vi "FinalProject_LastMinuteStuff.vi"() -> ()   [LabVIEW 2016]
uses:
  <vilib>/NXT/Block Support/NXT_TimerIndex.ctl
  <vilib>/NXT/Block Support/NXT_OutputPort.ctl
  <vilib>/NXT/Subs/ColorSensorColors.ctl
  <vilib>/NXT/Block Support/NXT_InputPort.ctl
  <vilib>/NXT/Dual Mode Library/Sensors/EV3_Color_Color.vi
  <vilib>/NXT/NXTIO Xnodes/NXTIONodeSubVIs/NXTMoveMotors.vi
  <vilib>/NXT/NXTIO Xnodes/NXTIONodeSubVIs/NXTStopMotors.vi
  <vilib>/NXT/NXTIO Xnodes/NXTIONodeSubVIs/NXTMotorRunDistance.vi
  <vilib>/NXT/Dual Mode Library/Sensors/EV3_Color_Reflect.vi
  <vilib>/NXT/Dual Mode Library/Waits/Wait_Num.vi
  <vilib>/NXT/Dual Mode Library/Sensors/Read_Timer.vi
  <vilib>/NXT/Dual Mode Library/Sensors/EV3_Color_RGB.vi
  <vilib>/NXT/Dual Mode Library/Sound/Tone.vi
  <vilib>/NXT/NXTIO Xnodes/AddressXNode/NXTIOAddress.xnode
  <vilib>/NXT/NXTIO Xnodes/NXTIOXNode/NXTIO.xnode
  <vilib>/NXT/Subs/LVHSConnector.ctl
  <vilib>/NXT/LegoClasses/BrickReference/BrickReference.lvclass
panel:
  out "Numeric 3":dbl
  out "Numeric 2":dbl
  out "Numeric":u32
  out "Process stopped":bool
  out "Red Large":i32
  out "Red Small":i32
  out "Blue Large":i32
  out "Blue Small":i32
  out "White Large":i32
  out "White Small":i32
  out "Steel":i32
  out "HDPE":i32
  out "Trash":i32
  out "1 Dose Small Pellets":i32
  out "1 Dose Large Pellets":i32
  out "Pellet Type":i32
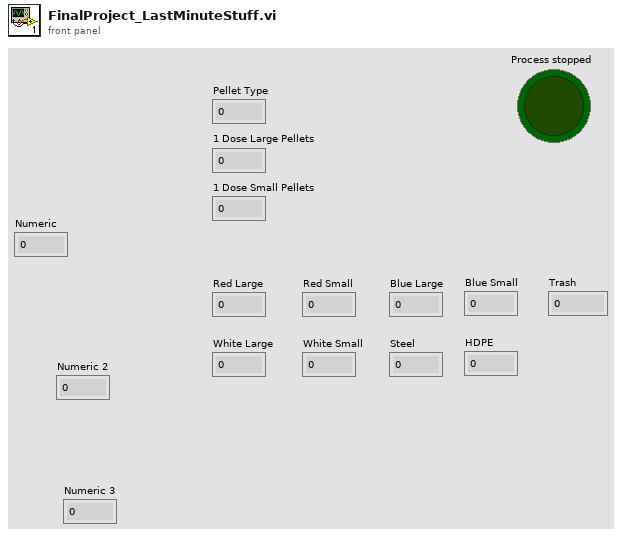
[diagram p1: front panel]
types:
  T1 = typedef "NXT_TimerIndex.ctl" = u8
  T2 = typedef "ColorSensorColors.ctl" = enum16{"No Color", "Black", "Blue", "Green", "Yellow", "Red", "White", "Brown"}
  T3 = typedef "NXT_InputPort.ctl" = u32
  T4 = typedef "NXT_OutputPort.ctl" = u8
  T5 = typedef "LVHSConnector.ctl" = refnum<class "BrickReference.lvclass">
  T6 = cluster{bool, bool, bool, bool, bool, bool, bool, bool}
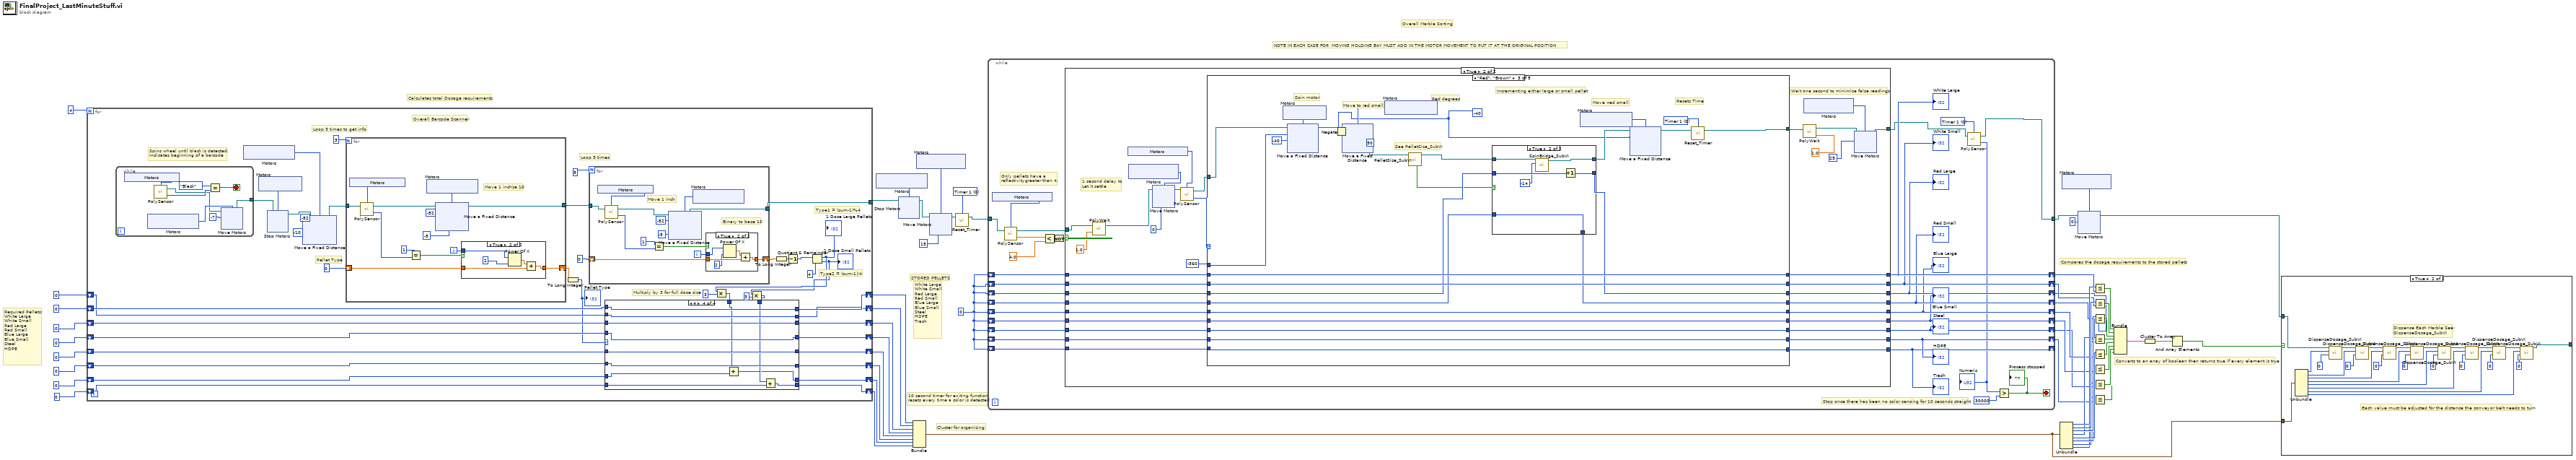
[diagram p0: block diagram]
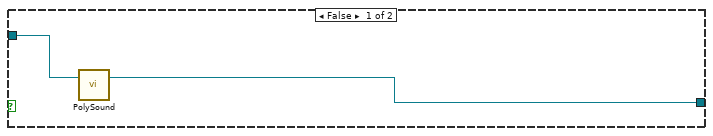
[diagram p2: hidden frame]
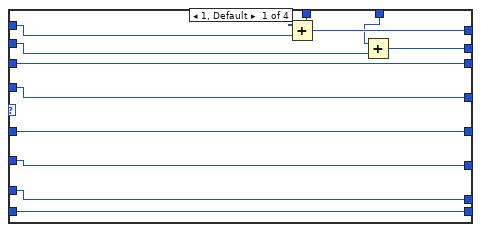
[diagram p3: hidden frame]
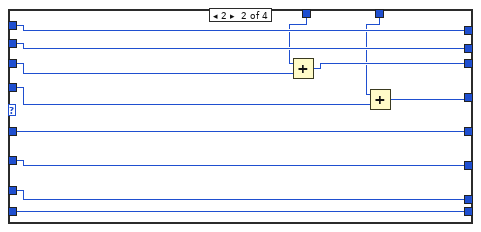
[diagram p4: hidden frame]
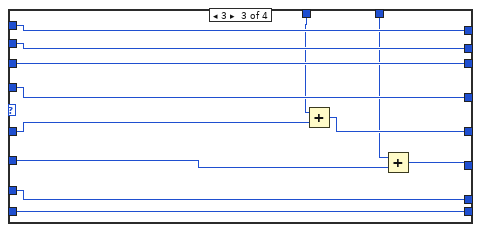
[diagram p5: hidden frame]
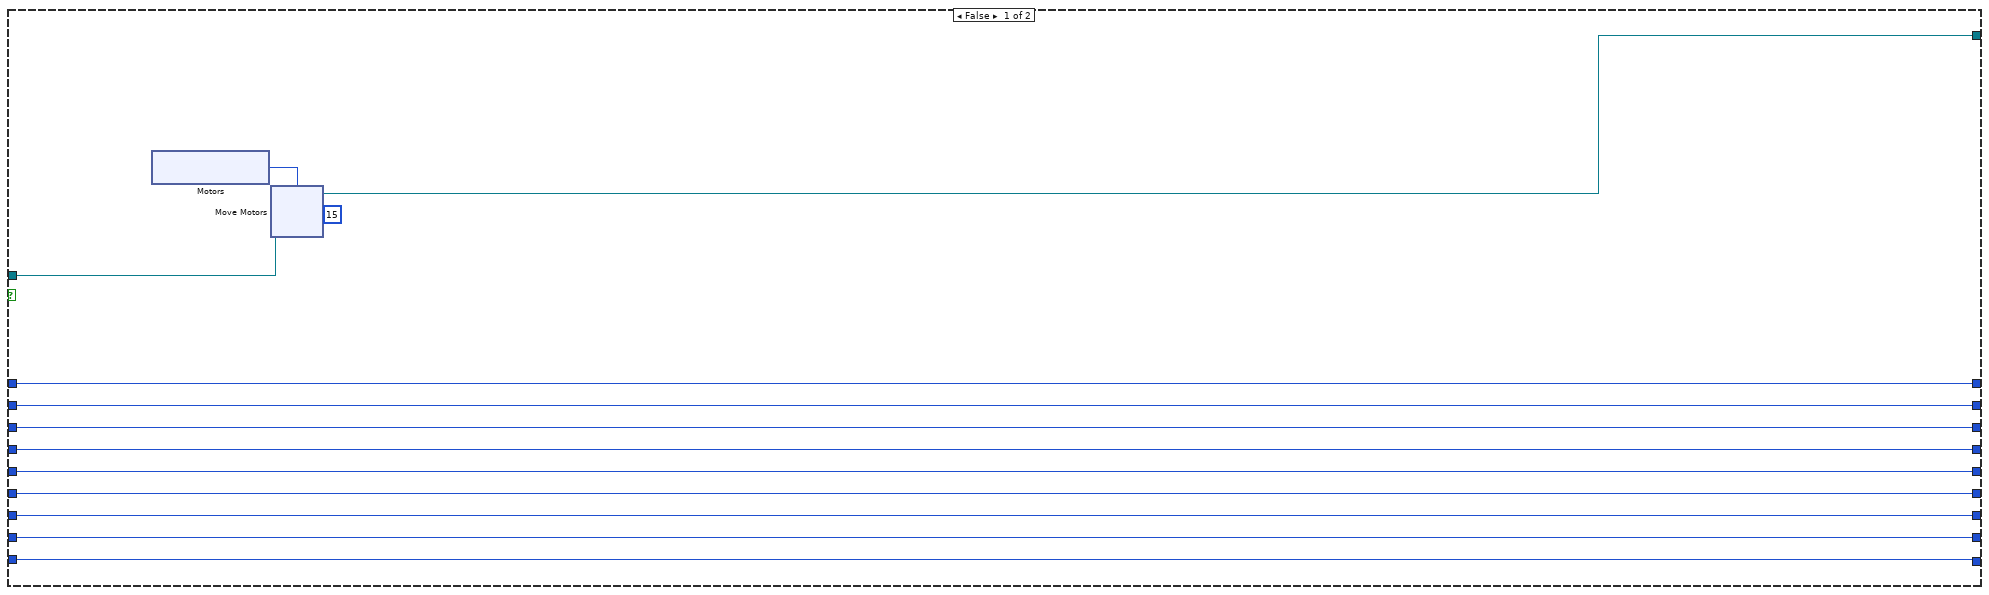
[diagram p8: hidden frame]
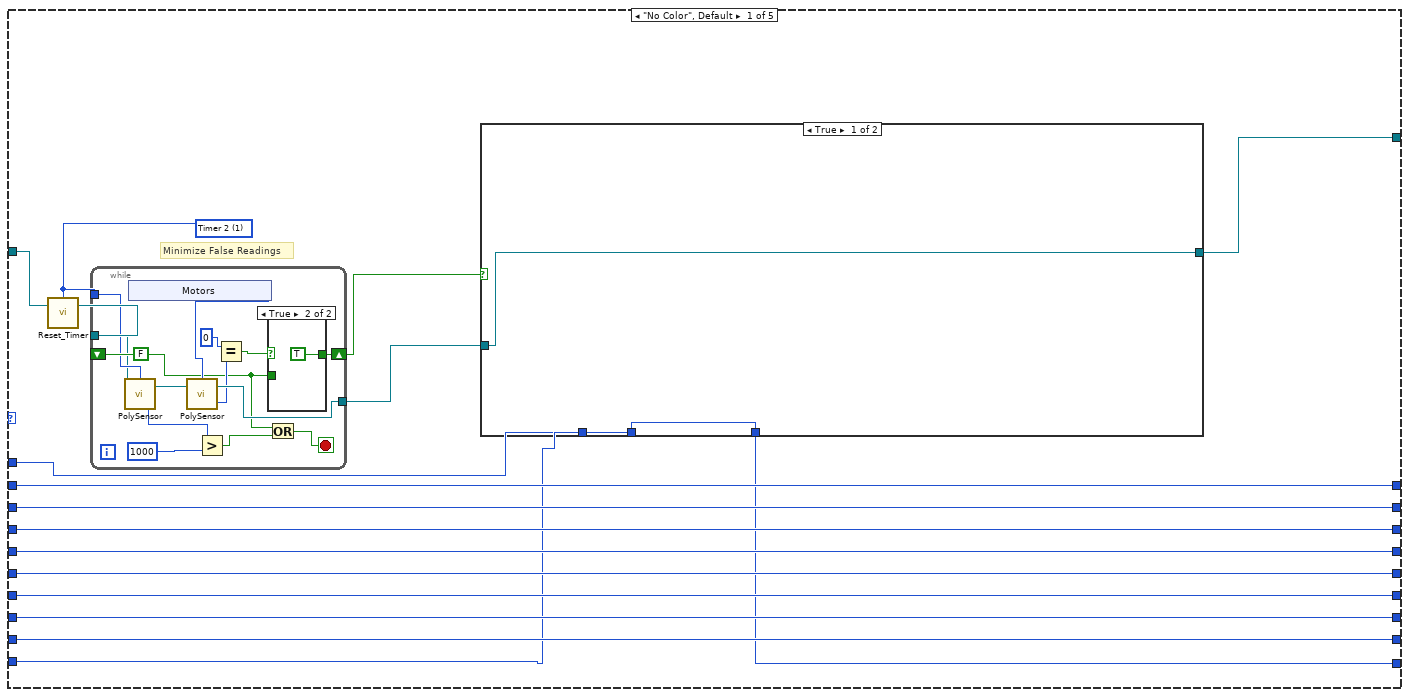
[diagram p9: hidden frame]
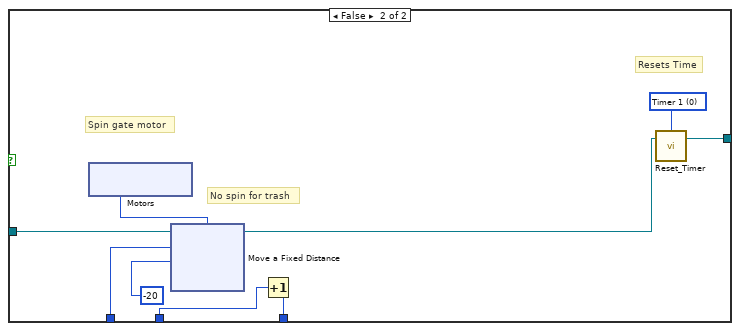
[diagram p10: hidden frame]
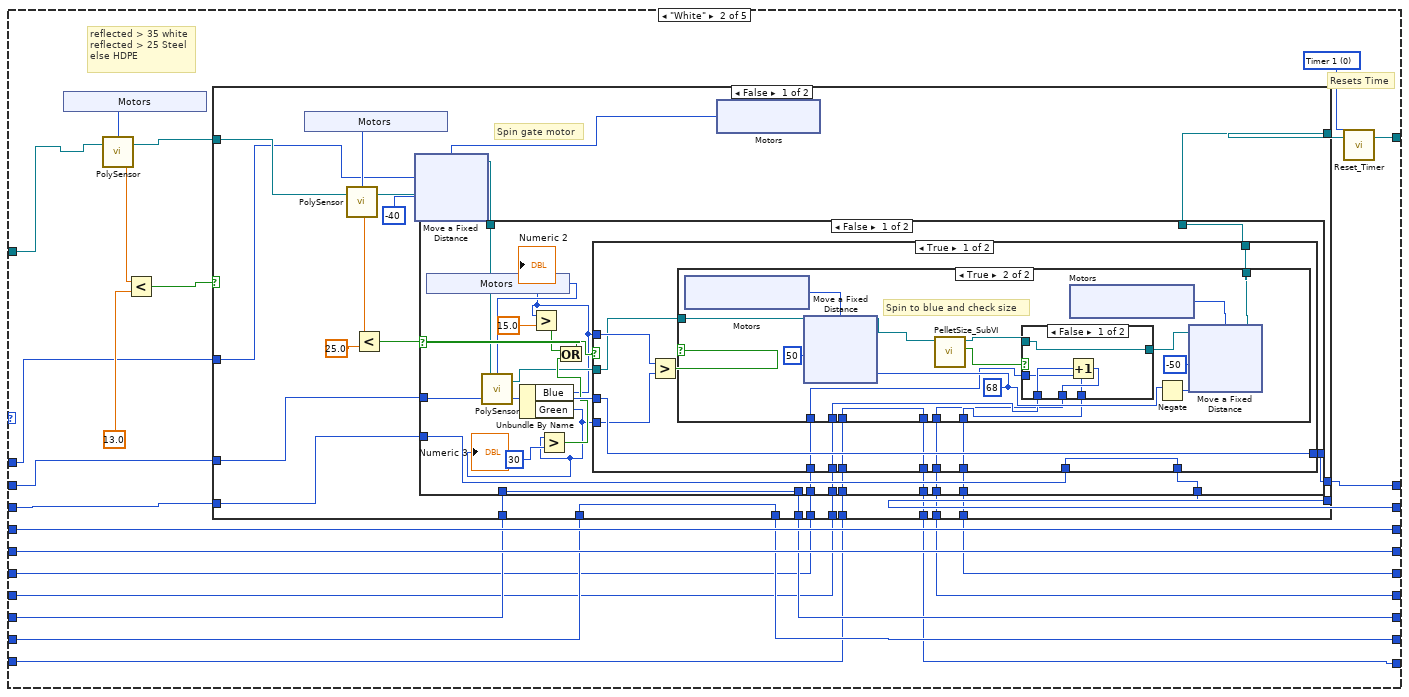
[diagram p12: hidden frame]
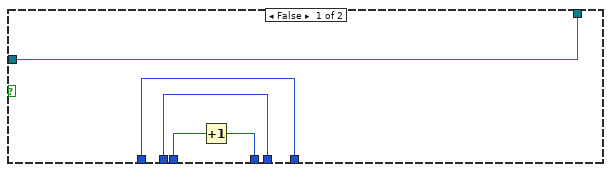
[diagram p13: hidden frame]
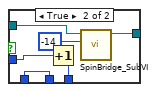
[diagram p14: hidden frame]
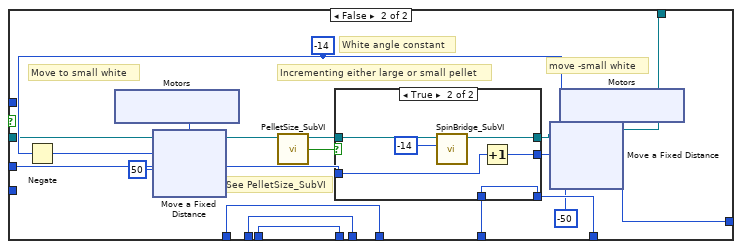
[diagram p15: hidden frame]
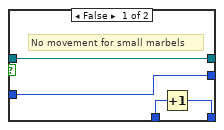
[diagram p16: hidden frame]
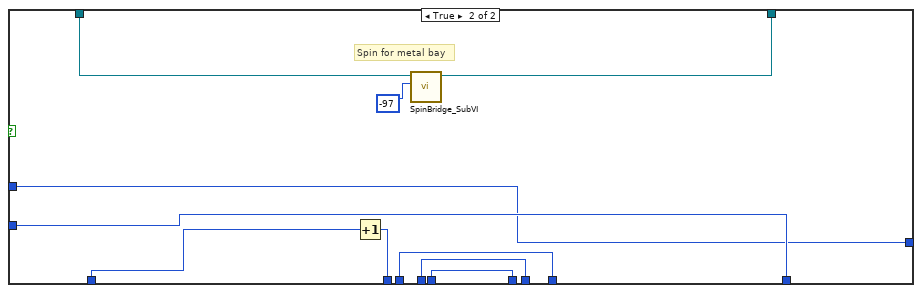
[diagram p17: hidden frame]
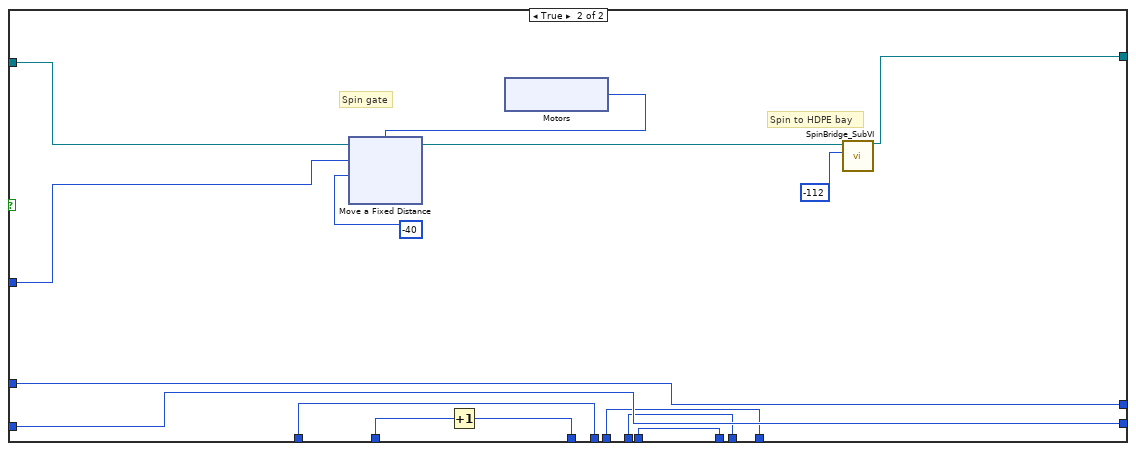
[diagram p18: hidden frame]
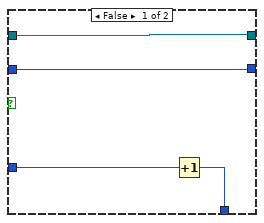
[diagram p19: hidden frame]
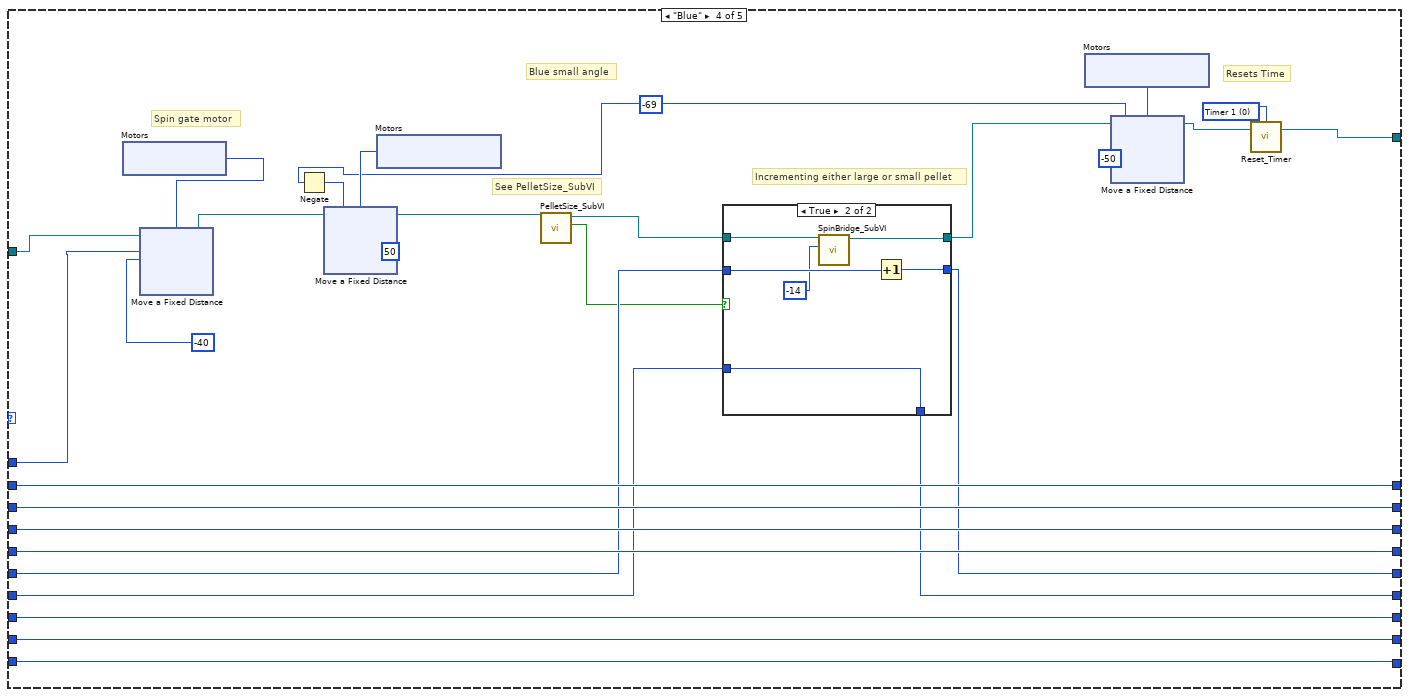
[diagram p20: hidden frame]
diagram:
  w11 = T1 0 items=["Timer 1", "Timer 2", "Timer 3"] ("Timer (Timer 1)")
  w12 = 0
  # "Cluster for organizing"
  # "Converts to an array of boolean then returns true if every element is true"
  # "Calculates total Dosage requirements"
  # "Compares the dosage requirements to the stored pellets"
  # "Required Pellets:\nWhite Large\nWhite Small\nRed Large\nRed Small\nBlue Large\nBlue Small\nSteel \nHDPE"
  # "STORED PELLETS"
  # "10 second timer for exiting function\nresets every time a color is detected"
  # "Overall Marble Sorting"
  # "NOTE IN EACH CASE FOR  MOVING HOLDING BAY MUST ADD IN THE MOTOR MOVEMENT TO PUT IT AT THE ORIGINAL POSITION"
  # "White Large\nWhite Small\nRed Large\nRed Small\nBlue Large\nBlue Small\nSteel\nHDPE\nTrash"
  n1 = for {
    N: 4 -> [_]
    tunnel: [w85] -> w14
    shift-right: [w70] -> w41
    shift-left: 0 -> [w84]
    shift-right: [w69] -> w40
    shift-left: 0 -> [w83]
    shift-right: [w76] -> w39
    shift-left: 0 -> [w82]
    shift-right: [w75] -> w38
    shift-left: 0 -> [w81]
    shift-right: [w74] -> w37
    shift-left: 0 -> [w80]
    shift-right: [w73] -> w36
    shift-left: 0 -> [w79]
    shift-right: [w72] -> w35
    shift-left: 0 -> [w78]
    shift-right: [w71] -> w17
    shift-left: 0 -> [w77]
    # "Multiply by 3 for full dose size"
    # "Overall Barcode Scanner"
    # "Spins wheel until black is detected.\nIndicates beginning of a barcode"
    # "Type2 = (sum-1)/4"
    # "Type1 = (sum-1)%4"
    # "Loop 5 times"
    # "Loop 3 times to get info"
    # "Pellet Type"
    n2 = while {
      tunnel: [w229] -> w99
      stop <- w230 stop-if-true
      n3 = xnode "Motors"() -> ("Sensor"=w227:T3)
      n4 = xnode "Motors"() -> ("Motor"=w233:T4)
      n5 = call-poly <vilib>:"PolySensor.vi"("Port (Port 1)"=w227) -> ("Detected Color"=w232:T2, "NXT/EV3"=w228:T5)  [unwired: 2 in]
      n6 = Equal?(x=ColorSensorColors."Black", y=w232) -> (x = y?=w230:bool)
      n7 = xnode "Move Motors"("Power/Speed 1"=i8 -7, "Motors"=w233, "NXT/EV3"=w228) -> ("NXT/EV3"=w229:T5)
    }
    n8 = xnode "Motors"() -> ("Motor"=w91:T4)
    n9 = xnode "Motors"() -> ("Motor"=w59:T4)
    n10 = xnode "Stop Motors"("Motors"=w59, "NXT/EV3"=w99) -> ("NXT/EV3"=w98:T5)
    n11 = xnode "Move a Fixed Distance"("Speed 1"=i8 -10, "Distance 1"=-52, "Motors"=w91, "NXT/EV3"=w98) -> ("NXT/EV3"=w96:T5)
    n12 = for {
      N: 3 -> [_]
      tunnel: w96 -> [w203]
      shift-right: [w197] -> w61
      shift-left: 0 -> [w200]
      tunnel: [w194] -> w87
      i -> [w201]
      # "Binary to base 10"
      # "Move 1 inch"
      n13 = xnode "Motors"() -> ("Sensor"=w191:T3)
      n14 = call-poly <vilib>:"PolySensor.vi"("NXT/EV3"=w203, "Port (Port 1)"=w191) -> ("Detected Color"=w202:T2, "NXT/EV3"=w199:T5)  [unwired: 1 in]
      n15 = Equal?(x=1, y=w202) -> (x = y?=w198:bool)
      n16 = xnode "Motors"() -> ("Motor"=w196:T4)
      n17 = xnode "Move a Fixed Distance"("Speed 1"=i8 -5, "Distance 1"=-52, "Motors"=w196, "NXT/EV3"=w199) -> ("NXT/EV3"=w194:T5)
      n18 = case shown="True" w198 {
        tunnel: w201 -> [_ w218]
        tunnel: w200 -> [w216 w220]
        tunnel: [w216 w219] -> w197
        frame False {
        }
        frame True {
          n19 = Power Of X(1:2, 2:w218) -> (0:w221:dbl)
          n20 = Add(x=w221, y=w220) -> (x+y=w219:dbl)
        }
      }
    }
    n21 = To Long Integer(number=w61) -> (32bit integer=w60:i32)
    "Pellet Type" <- w60
    n22 = for {
      N: 5 -> [_]
      shift-right: [w158] -> w90
      shift-left: 0 -> [w155]
      tunnel: [w157] -> w85
      tunnel: w87 -> [w156]
      i -> [w161]
      # "Binary to base 10"
      # "Move 1 inch"
      n23 = xnode "Motors"() -> ("Sensor"=w150:T3)
      n24 = call-poly <vilib>:"PolySensor.vi"("NXT/EV3"=w156, "Port (Port 1)"=w150) -> ("Detected Color"=w162:T2, "NXT/EV3"=w160:T5)  [unwired: 1 in]
      n25 = Equal?(x=1, y=w162) -> (x = y?=w159:bool)
      n26 = xnode "Motors"() -> ("Motor"=w154:T4)
      n27 = xnode "Move a Fixed Distance"("Speed 1"=i8 -5, "Distance 1"=-52, "Motors"=w154, "NXT/EV3"=w160) -> ("NXT/EV3"=w157:T5)
      n28 = case shown="True" w159 {
        tunnel: w161 -> [_ w176]
        tunnel: w155 -> [w175 w179]
        tunnel: [w175 w178] -> w158
        frame False {
        }
        frame True {
          n29 = Power Of X(1:2, 2:w176) -> (0:w180:dbl)
          n30 = Add(x=w180, y=w179) -> (x+y=w178:dbl)
        }
      }
    }
    n31 = To Long Integer(number=w90) -> (32bit integer=w89:i32)
    n32 = Decrement(x=w89) -> (x-1=w68:i32)
    n33 = Quotient & Remainder(x=w68, y=4) -> (x-y*floor(x/y)=w65:i32, floor(x/y)=w63:i32)
    "1 Dose Small Pellets" <- w63
    "1 Dose Large Pellets" <- w65
    n34 = Multiply(x=w65, y=3) -> (x*y=w64:i32)
    n35 = Multiply(x=w63, y=3) -> (x*y=w62:i32)
    n36 = case shown="4" w60 {
      tunnel: w84 -> [w105 w124 w136 w148]
      tunnel: w83 -> [w103 w123 w135 w147]
      tunnel: w82 -> [w112 w117 w134 w146]
      tunnel: w81 -> [w111 w115 w133 w145]
      tunnel: w80 -> [w110 w122 w127 w144]
      tunnel: w79 -> [w109 w121 w128 w143]
      tunnel: w78 -> [w108 w120 w126 w139]
      tunnel: w77 -> [w107 w119 w125 w138]
      tunnel: w64 -> [w106 w118 w132 w142]
      tunnel: w62 -> [w102 w114 w130 w141]
      tunnel: [w112 w116 w134 w146] -> w76
      tunnel: [w111 w113 w133 w145] -> w75
      tunnel: [w110 w122 w131 w144] -> w74
      tunnel: [w109 w121 w129 w143] -> w73
      tunnel: [w108 w120 w126 w140] -> w72
      tunnel: [w107 w119 w125 w137] -> w71
      tunnel: [w104 w124 w136 w148] -> w70
      tunnel: [w101 w123 w135 w147] -> w69
      frame 1, Default {
        n37 = Add(x=w106, y=w105) -> (x+y=w104:i32)
        n38 = Add(x=w102, y=w103) -> (x+y=w101:i32)
      }
      frame 2 {
        n39 = Add(x=w118, y=w117) -> (x+y=w116:i32)
        n40 = Add(x=w114, y=w115) -> (x+y=w113:i32)
      }
      frame 3 {
        n41 = Add(x=w132, y=w127) -> (x+y=w131:i32)
        n42 = Add(x=w130, y=w128) -> (x+y=w129:i32)
      }
      frame 4 {
        n43 = Add(x=w142, y=w139) -> (x+y=w140:i32)
        n44 = Add(x=w141, y=w138) -> (x+y=w137:i32)
      }
    }
  }
  n45 = xnode "Motors"() -> ("Motor"=w13:T4)
  n46 = xnode "Stop Motors"("Motors"=w13, "NXT/EV3"=w14) -> ("NXT/EV3"=w8:T5)
  n47 = Bundle(w41, w40, w39, w38, w37, w36, w35, w17) -> (w10:cluster{i32, i32, i32, i32, i32, i32, i32, i32})  [unwired: 1 in]
  n48 = xnode "Motors"() -> ("Motor"=w9:T4)
  n49 = xnode "Move Motors"("Power/Speed 1"=i8 15, "Motors"=w9, "NXT/EV3"=w8) -> ("NXT/EV3"=w7:T5)
  n50 = call <vilib>:"Reset_Timer.vi"("NXT/EV3"=w7, "Timer (Timer 1)"=w11) -> ("NXT/EV3"=w5:T5)  [unwired: 2 in]
  n51 = while {
    shift-right: [w260] -> w26
    shift-left: w12 -> [w269]
    shift-right: [w259] -> w25
    shift-left: w12 -> [w268]
    shift-right: [w258] -> w24
    shift-left: w12 -> [w267]
    shift-right: [w257] -> w23
    shift-left: w12 -> [w266]
    shift-right: [w254] -> w22
    shift-left: w12 -> [w265]
    shift-right: [w253] -> w21
    shift-left: w12 -> [w264]
    shift-right: [w252] -> w20
    shift-left: w12 -> [w263]
    shift-right: [w256] -> w19
    shift-left: w12 -> [w262]
    shift-right: [w255] -> _
    shift-left: w12 -> [w261]
    tunnel: w5 -> [w245]
    tunnel: [w244] -> w3
    stop <- w249 stop-if-true
    w247 = T1 0 items=["Timer 1", "Timer 2", "Timer 3"] ("Timer (Timer 1)")
    # "Stop once there has been no color sensing for 10 seconds straight"
    # "Only pellets have a\nreflectivitygreater than 4."
    n52 = xnode "Motors"() -> ("Sensor"=w251:T3)
    n53 = call-poly <vilib>:"PolySensor.vi"("NXT/EV3"=w245, "Port (Port 1)"=w251) -> ("Scaled Value"=w274:sgl, "NXT/EV3"=w270:T5)  [unwired: 1 in]
    n54 = Less?(x=w274, y=sgl 4.0) -> (x < y?=w273:bool)
    n55 = Not(x=w273) -> (.not. x?=w271:bool)
    n56 = case shown="True" w271 {
      tunnel: w270 -> [w277 w305]
      tunnel: w269 -> [w288 w329]
      tunnel: w268 -> [w287 w328]
      tunnel: w267 -> [w286 w327]
      tunnel: w266 -> [w285 w326]
      tunnel: w265 -> [w284 w325]
      tunnel: w264 -> [w283 w324]
      tunnel: w263 -> [w282 w323]
      tunnel: w262 -> [w281 w322]
      tunnel: w261 -> [w280 w321]
      tunnel: [w280 w320] -> w255
      tunnel: [w281 w318] -> w256
      tunnel: [w282 w317] -> w252
      tunnel: [w283 w316] -> w253
      tunnel: [w285 w315] -> w257
      tunnel: [w284 w314] -> w254
      tunnel: [w286 w313] -> w258
      tunnel: [w288 w312] -> w260
      tunnel: [w287 w311] -> w259
      tunnel: [w276 w300] -> w248
      frame False {
        n57 = xnode "Motors"() -> ("Motor"=w279:T4)
        n58 = xnode "Move Motors"("Power/Speed 1"=i8 15, "Motors"=w279, "NXT/EV3"=w277) -> ("NXT/EV3"=w276:T5)
      }
      frame True {
        # "Wait one second to minimize false readings"
        # "1 second delay to\nLet it settle"
        n59 = call-poly <vilib>:"PolyWait.vi"("Time (1 sec)"=sgl 1.0, "NXT/EV3"=w305) -> ("NXT/EV3"=w303:T5)  [unwired: 2 in]
        n60 = xnode "Motors"() -> ("Sensor"=w310:T3)
        n61 = xnode "Motors"() -> ("Motor"=w302:T4)
        n62 = xnode "Move Motors"("Power/Speed 1"=i8 0, "Motors"=w302, "NXT/EV3"=w303) -> ("NXT/EV3"=w307:T5)
        n63 = call-poly <vilib>:"PolySensor.vi"("NXT/EV3"=w307, "Port (Port 1)"=w310) -> ("Detected Color"=w319:T2, "NXT/EV3"=w330:T5)  [unwired: 1 in]
        n64 = case shown="\"Red\", \"Brown\"" w319 {
          tunnel: w330 -> [w352 w412 w660 w733 w794]
          tunnel: w329 -> [w359 w417 w673 w745 w803]
          tunnel: w328 -> [w358 w423 w672 w744 w802]
          tunnel: w327 -> [w360 w430 w666 w743 w801]
          tunnel: w326 -> [w362 w429 w665 w742 w800]
          tunnel: w325 -> [w361 w405 w671 w741 w799]
          tunnel: w324 -> [w363 w407 w670 w740 w798]
          tunnel: w323 -> [w364 w424 w669 w737 w797]
          tunnel: w322 -> [w365 w425 w668 w736 w806]
          tunnel: w321 -> [w350 w409 w667 w735 w807]
          tunnel: [w349 w410 w667 w735 w804] -> w320
          tunnel: [w357 w413 w649 w721 w796] -> w309
          tunnel: [w365 w422 w668 w736 w805] -> w318
          tunnel: [w364 w421 w669 w737 w797] -> w317
          tunnel: [w363 w408 w670 w738 w798] -> w316
          tunnel: [w362 w429 w663 w742 w800] -> w315
          tunnel: [w361 w406 w671 w739 w799] -> w314
          tunnel: [w360 w430 w664 w743 w801] -> w313
          tunnel: [w359 w419 w673 w745 w803] -> w312
          tunnel: [w358 w420 w672 w744 w802] -> w311
          tunnel: -360 -> [w348 w411 w646 w718 w789]
          frame "No Color", Default {
            w356 = T1 1 items=["Timer 1", "Timer 2", "Timer 3"] ("Timer (Timer 1)")
            # "Minimize False Readings"
            n65 = call <vilib>:"Reset_Timer.vi"("NXT/EV3"=w352, "Timer (Timer 1)"=w356) -> ("NXT/EV3"=w355:T5)  [unwired: 2 in]
            n66 = while {
              tunnel: w356 -> [w401]
              tunnel: w355 -> [w400]
              tunnel: [w395] -> w353
              shift-right: [w397] -> w351
              shift-left: FALSE -> [w389]
              stop <- w388 stop-if-true
              n67 = call-poly <vilib>:"PolySensor.vi"("NXT/EV3"=w400, "Timer (Timer 1)"=w401) -> ("Value (msec)"=w398:u32, "NXT/EV3"=w396:T5)  [unwired: 1 in]
              n68 = xnode "Motors"() -> ("Sensor"=w391:T3)
              n69 = call-poly <vilib>:"PolySensor.vi"("NXT/EV3"=w396, "Port (Port 1)"=w391) -> ("Detected Color"=w393:T2, "NXT/EV3"=w395:T5)  [unwired: 1 in]
              n70 = Greater?(x=w398, y=u32 1000) -> (0:w390:bool)
              n71 = Equal?(x=0, y=w393) -> (x = y?=w392:bool)
              n72 = case shown="True" w392 {
                tunnel: [w403 TRUE] -> w397
                tunnel: w389 -> [w403 _]
                frame False {
                }
                frame True {
                }
              }
              n73 = Or(x=w389, y=w390) -> (x .or. y?=w388:bool)
            }
            n74 = case shown="True" w351 {
              tunnel: [w367 w373] -> w357
              tunnel: w353 -> [w367 w371]
              tunnel: w350 -> [w366 w370]
              tunnel: [w366 w369] -> w349
              tunnel: w348 -> [_ w368]
              frame True {
              }
              frame False {
                w372 = T1 0 items=["Timer 1", "Timer 2", "Timer 3"] ("Timer (Timer 1)")
                # "Resets Time"
                # "No spin for trash"
                # "Spin gate motor"
                n75 = xnode "Motors"() -> ("Motor"=w376:T4)
                n76 = xnode "Move a Fixed Distance"("Speed 1"=i8 -20, "Distance 1"=w368, "Motors"=w376, "NXT/EV3"=w371) -> ("NXT/EV3"=w374:T5)
                n77 = Increment(x=w370) -> (x+1=w369:i32)
                n78 = call <vilib>:"Reset_Timer.vi"("NXT/EV3"=w374, "Timer (Timer 1)"=w372) -> ("NXT/EV3"=w373:T5)  [unwired: 2 in]
              }
            }
          }
          frame "White" {
            w414 = T1 0 items=["Timer 1", "Timer 2", "Timer 3"] ("Timer (Timer 1)")
            # "Resets Time"
            # "reflected > 35 white\nreflected > 25 Steel\nelse HDPE"
            n79 = xnode "Motors"() -> ("Sensor"=w416:T3)
            n80 = call-poly <vilib>:"PolySensor.vi"("NXT/EV3"=w412, "Port (Port 1)"=w416) -> ("Scaled Value"=w428:sgl, "NXT/EV3"=w418:T5)  [unwired: 1 in]
            n81 = Less?(x=w428, y=sgl 13.0) -> (x < y?=w426:bool)
            n82 = case shown="False" w426 {
              tunnel: w425 -> [w455 w634]
              tunnel: w424 -> [w453 w632]
              tunnel: w423 -> [w449 w631]
              tunnel: w417 -> [w445 w630]
              tunnel: [w455 w633] -> w422
              tunnel: [w448 w632] -> w421
              tunnel: [w447 w631] -> w420
              tunnel: [w446 w630] -> w419
              tunnel: w418 -> [w454 w627]
              tunnel: [w444 w625] -> w415
              tunnel: w411 -> [w438 w623]
              tunnel: [w437 w622] -> w410
              tunnel: w409 -> [w436 w622]
              tunnel: [w435 w621] -> w408
              tunnel: w407 -> [w434 w621]
              tunnel: [w433 w620] -> w406
              tunnel: w405 -> [w432 w620]
              frame False {
                # "Spin gate motor"
                n83 = xnode "Motors"() -> ("Sensor"=w443:T3)
                n84 = call-poly <vilib>:"PolySensor.vi"("NXT/EV3"=w454, "Port (Port 1)"=w443) -> ("Scaled Value"=w452:sgl, "NXT/EV3"=w440:T5)  [unwired: 1 in]
                n85 = Less?(x=w452, y=sgl 25.0) -> (x < y?=w450:bool)
                n86 = xnode "Motors"() -> ("Motor"=w442:T4)
                n87 = xnode "Move a Fixed Distance"("Speed 1"=i8 -40, "Distance 1"=w438, "Motors"=w442, "NXT/EV3"=w440) -> ("NXT/EV3"=w439:T5)
                n88 = case shown="False" w450 {
                  tunnel: w453 -> [w490 w616]
                  tunnel: w449 -> [w489 w618]
                  tunnel: w445 -> [w487 w617]
                  tunnel: [w490 w619] -> w448
                  tunnel: [w488 w618] -> w447
                  tunnel: [w486 w617] -> w446
                  tunnel: [w485 w614] -> w444
                  tunnel: w439 -> [w484 w615]
                  tunnel: [w480 w612] -> w437
                  tunnel: w436 -> [w479 w612]
                  tunnel: [w473 w611] -> w435
                  tunnel: w434 -> [w472 w611]
                  tunnel: [w471 w610] -> w433
                  tunnel: w432 -> [w470 w610]
                  frame False {
                    n89 = xnode "Motors"() -> ("Sensor"=w483:T3)
                    n90 = call-poly <vilib>:"PolySensor.vi"("NXT/EV3"=w484, "Port (Port 1)"=w483) -> ("RGB Color"=w482:cluster{"Red":u8, "Green":u8, "Blue":u8}, "NXT/EV3"=w474:T5)  [unwired: 1 in]
                    n91 = Unbundle By Name(w482) -> ("Blue"=w468:u8, "Green"=w469:u8)
                    "Numeric 2" <- w468
                    "Numeric 3" <- w469
                    n92 = Greater?(x=w468, y=15.0) -> (0:w477:bool)
                    n93 = Greater?(x=w469, y=30) -> (0:w476:bool)
                    n94 = Or(x=w477, y=w476) -> (x .or. y?=w475:bool)
                    n95 = case shown="True" w475 {
                      tunnel: w489 -> [w502 w576]
                      tunnel: [w502 w575] -> w488
                      tunnel: w487 -> [w503 w574]
                      tunnel: [w503 w573] -> w486
                      tunnel: [w492 w568] -> w485
                      tunnel: [w500 w561] -> w480
                      tunnel: w479 -> [w501 w561]
                      tunnel: w474 -> [w491 w560]
                      tunnel: [w499 w559] -> w473
                      tunnel: w472 -> [w498 w559]
                      tunnel: w469 -> [w497 _]
                      tunnel: w468 -> [w496 _]
                      tunnel: [w494 w558] -> w471
                      tunnel: w470 -> [w493 w558]
                      frame True {
                        n96 = Greater?(x=w496, y=w497) -> (0:w495:bool)
                        n97 = case shown="True" w495 {
                          tunnel: w501 -> [w508 w525]
                          tunnel: [w507 w525] -> w500
                          tunnel: [w506 w511] -> w499
                          tunnel: w498 -> [w506 w514]
                          tunnel: [w505 w512] -> w494
                          tunnel: w493 -> [w505 w513]
                          tunnel: [w504 w520] -> w492
                          tunnel: w491 -> [w504 w523]
                          frame False {
                            n98 = Increment(x=w508) -> (x+1=w507:i32)
                          }
                          frame True {
                            w519 = 68
                            # "Spin to blue and check size"
                            n99 = xnode "Motors"() -> ("Motor"=w522:T4)
                            n100 = xnode "Move a Fixed Distance"("Speed 1"=i8 50, "Distance 1"=w519, "Motors"=w522, "NXT/EV3"=w523) -> ("NXT/EV3"=w516:T5)
                            n101 = call "PelletSize_SubVI.vi"("BrickReference in"=w516) -> ("Boolean"=w524:bool, "BrickReference out"=w510:T5)  [unwired: 9 in]
                            n102 = case shown="False" w524 {
                              tunnel: w514 -> [w541 w545]
                              tunnel: w513 -> [w539 w547]
                              tunnel: [w539 w546] -> w512
                              tunnel: [w540 w545] -> w511
                              tunnel: w510 -> [w538 w543]
                              tunnel: [w538 w542] -> w509
                              frame False {
                                n103 = Increment(x=w541) -> (x+1=w540:i32)
                              }
                              frame True {
                                n104 = Increment(x=w547) -> (x+1=w546:i32)
                                n105 = call "SpinBridge_SubVI.vi"("Motor Spin in"=-14, "BrickReference in"=w543) -> ("BrickReference out"=w542:T5)  [unwired: 9 in]
                              }
                            }
                            n106 = xnode "Motors"() -> ("Motor"=w521:T4)
                            n107 = Negate(x=w519) -> (-x=w518:i32)
                            n108 = xnode "Move a Fixed Distance"("Speed 1"=i8 -50, "Distance 1"=w518, "Motors"=w521, "NXT/EV3"=w509) -> ("NXT/EV3"=w520:T5)
                          }
                        }
                      }
                      frame False {
                        w563 = -14
                        # "White angle constant"
                        # "move -small white"
                        # "Move to small white"
                        # "See PelletSize_SubVI"
                        # "Incrementing either large or small pellet"
                        n109 = Negate(x=w563) -> (-x=w567:i32)
                        n110 = xnode "Motors"() -> ("Motor"=w565:T4)
                        n111 = xnode "Move a Fixed Distance"("Speed 1"=i8 50, "Distance 1"=w567, "Motors"=w565, "NXT/EV3"=w560) -> ("NXT/EV3"=w570:T5)
                        n112 = call "PelletSize_SubVI.vi"("BrickReference in"=w570) -> ("Boolean"=w572:bool, "BrickReference out"=w571:T5)  [unwired: 9 in]
                        n113 = case shown="True" w572 {
                          tunnel: w576 -> [w602 w608]
                          tunnel: [w601 w608] -> w575
                          tunnel: w574 -> [w600 w607]
                          tunnel: [w600 w606] -> w573
                          tunnel: w571 -> [w599 w605]
                          tunnel: [w599 w604] -> w569
                          frame False {
                            # "No movement for small marbels"
                            n114 = Increment(x=w602) -> (x+1=w601:i32)
                          }
                          frame True {
                            n115 = call "SpinBridge_SubVI.vi"("Motor Spin in"=-14, "BrickReference in"=w605) -> ("BrickReference out"=w604:T5)  [unwired: 9 in]
                            n116 = Increment(x=w607) -> (x+1=w606:i32)
                          }
                        }
                        n117 = xnode "Motors"() -> ("Motor"=w564:T4)
                        n118 = xnode "Move a Fixed Distance"("Speed 1"=i8 -50, "Distance 1"=w563, "Motors"=w564, "NXT/EV3"=w569) -> ("NXT/EV3"=w568:T5)
                      }
                    }
                  }
                  frame True {
                    # "Spin for metal bay"
                    n119 = Increment(x=w616) -> (x+1=w619:i32)
                    n120 = call "SpinBridge_SubVI.vi"("Motor Spin in"=-97, "BrickReference in"=w615) -> ("BrickReference out"=w614:T5)  [unwired: 9 in]
                  }
                }
              }
              frame True {
                # "Spin to HDPE bay"
                # "Spin gate"
                n121 = Increment(x=w634) -> (x+1=w633:i32)
                n122 = xnode "Motors"() -> ("Motor"=w629:T4)
                n123 = xnode "Move a Fixed Distance"("Speed 1"=i8 -40, "Distance 1"=w623, "Motors"=w629, "NXT/EV3"=w627) -> ("NXT/EV3"=w626:T5)
                n124 = call "SpinBridge_SubVI.vi"("Motor Spin in"=-112, "BrickReference in"=w626) -> ("BrickReference out"=w625:T5)  [unwired: 9 in]
              }
            }
            n125 = call <vilib>:"Reset_Timer.vi"("NXT/EV3"=w415, "Timer (Timer 1)"=w414) -> ("NXT/EV3"=w413:T5)  [unwired: 2 in]
          }
          frame "Red", "Brown" {
            w648 = T1 0 items=["Timer 1", "Timer 2", "Timer 3"] ("Timer (Timer 1)")
            w647 = -40
            # "Resets Time"
            # "Red degrees"
            # "Move -red small"
            # "Move to red small"
            # "See PelletSize_SubVI"
            # "Incrementing either large or small pellet"
            # "Spin motor"
            n126 = xnode "Motors"() -> ("Motor"=w662:T4)
            n127 = xnode "Move a Fixed Distance"("Speed 1"=i8 -40, "Distance 1"=w646, "Motors"=w662, "NXT/EV3"=w660) -> ("NXT/EV3"=w656:T5)
            n128 = Negate(x=w647) -> (-x=w654:i32)
            n129 = xnode "Motors"() -> ("Motor"=w652:T4)
            n130 = xnode "Move a Fixed Distance"("Speed 1"=i8 50, "Distance 1"=w654, "Motors"=w652, "NXT/EV3"=w656) -> ("NXT/EV3"=w657:T5)
            n131 = call "PelletSize_SubVI.vi"("BrickReference in"=w657) -> ("Boolean"=w658:bool, "BrickReference out"=w659:T5)  [unwired: 9 in]
            n132 = case shown="True" w658 {
              tunnel: w666 -> [w710 w716]
              tunnel: w665 -> [w709 w714]
              tunnel: [w710 w715] -> w664
              tunnel: [w708 w714] -> w663
              tunnel: w659 -> [w707 w713]
              tunnel: [w707 w712] -> w655
              frame False {
                n133 = Increment(x=w709) -> (x+1=w708:i32)
              }
              frame True {
                n134 = call "SpinBridge_SubVI.vi"("Motor Spin in"=-14, "BrickReference in"=w713) -> ("BrickReference out"=w712:T5)  [unwired: 9 in]
                n135 = Increment(x=w716) -> (x+1=w715:i32)
              }
            }
            n136 = xnode "Motors"() -> ("Motor"=w651:T4)
            n137 = xnode "Move a Fixed Distance"("Speed 1"=w647, "Distance 1"=w647, "Motors"=w651, "NXT/EV3"=w655) -> ("NXT/EV3"=w650:T5)
            n138 = call <vilib>:"Reset_Timer.vi"("NXT/EV3"=w650, "Timer (Timer 1)"=w648) -> ("NXT/EV3"=w649:T5)  [unwired: 2 in]
          }
          frame "Blue" {
            w720 = T1 0 items=["Timer 1", "Timer 2", "Timer 3"] ("Timer (Timer 1)")
            w719 = -69
            # "Resets Time"
            # "Blue small angle"
            # "See PelletSize_SubVI"
            # "Incrementing either large or small pellet"
            # "Spin gate motor"
            n139 = xnode "Motors"() -> ("Motor"=w730:T4)
            n140 = xnode "Move a Fixed Distance"("Speed 1"=i8 -40, "Distance 1"=w718, "Motors"=w730, "NXT/EV3"=w733) -> ("NXT/EV3"=w729:T5)
            n141 = Negate(x=w719) -> (-x=w726:i32)
            n142 = xnode "Motors"() -> ("Motor"=w724:T4)
            n143 = xnode "Move a Fixed Distance"("Speed 1"=i8 50, "Distance 1"=w726, "Motors"=w724, "NXT/EV3"=w729) -> ("NXT/EV3"=w728:T5)
            n144 = call "PelletSize_SubVI.vi"("BrickReference in"=w728) -> ("Boolean"=w732:bool, "BrickReference out"=w731:T5)  [unwired: 9 in]
            n145 = case shown="True" w732 {
              tunnel: w741 -> [w782 w788]
              tunnel: w740 -> [w781 w786]
              tunnel: [w782 w787] -> w739
              tunnel: [w780 w786] -> w738
              tunnel: w731 -> [w779 w785]
              tunnel: [w779 w784] -> w727
              frame False {
                n146 = Increment(x=w781) -> (x+1=w780:i32)
              }
              frame True {
                n147 = call "SpinBridge_SubVI.vi"("Motor Spin in"=-14, "BrickReference in"=w785) -> ("BrickReference out"=w784:T5)  [unwired: 9 in]
                n148 = Increment(x=w788) -> (x+1=w787:i32)
              }
            }
            n149 = xnode "Motors"() -> ("Motor"=w723:T4)
            n150 = xnode "Move a Fixed Distance"("Speed 1"=-50, "Distance 1"=w719, "Motors"=w723, "NXT/EV3"=w727) -> ("NXT/EV3"=w722:T5)
            n151 = call <vilib>:"Reset_Timer.vi"("NXT/EV3"=w722, "Timer (Timer 1)"=w720) -> ("NXT/EV3"=w721:T5)  [unwired: 2 in]
          }
          frame "Black" {
            w795 = T1 1 items=["Timer 1", "Timer 2", "Timer 3"] ("Timer (Timer 1)")
            # "Minimize False Readings"
            n152 = call <vilib>:"Reset_Timer.vi"("NXT/EV3"=w794, "Timer (Timer 1)"=w795) -> ("NXT/EV3"=w793:T5)  [unwired: 2 in]
            n153 = while {
              tunnel: w795 -> [w821]
              tunnel: w793 -> [w820]
              tunnel: [w815] -> w792
              shift-right: [w817] -> w790
              shift-left: FALSE -> [w809]
              stop <- w808 stop-if-true
              n154 = call-poly <vilib>:"PolySensor.vi"("NXT/EV3"=w820, "Timer (Timer 1)"=w821) -> ("Value (msec)"=w818:u32, "NXT/EV3"=w816:T5)  [unwired: 1 in]
              n155 = xnode "Motors"() -> ("Sensor"=w811:T3)
              n156 = call-poly <vilib>:"PolySensor.vi"("NXT/EV3"=w816, "Port (Port 1)"=w811) -> ("Detected Color"=w813:T2, "NXT/EV3"=w815:T5)  [unwired: 1 in]
              n157 = Greater?(x=w818, y=u32 1000) -> (0:w810:bool)
              n158 = Equal?(x=0, y=w813) -> (x = y?=w812:bool)
              n159 = case shown="True" w812 {
                tunnel: [w823 TRUE] -> w817
                tunnel: w809 -> [w823 _]
                frame False {
                }
                frame True {
                }
              }
              n160 = Or(x=w809, y=w810) -> (x .or. y?=w808:bool)
            }
            n161 = case shown="False" w790 {
              tunnel: w807 -> [w838 w866]
              tunnel: w806 -> [w837 w865]
              tunnel: [w836 w865] -> w805
              tunnel: [w835 w866] -> w804
              tunnel: w792 -> [w834 w864]
              tunnel: [w827 w864] -> w796
              tunnel: w789 -> [w825 _]
              frame False {
                w826 = T1 0 items=["Timer 1", "Timer 2", "Timer 3"] ("Timer (Timer 1)")
                # "Resets Time"
                # "Determine if a trash or opaque pellet"
                # "Spin gate"
                # "if reflect > 15 HDPE\nelse trash"
                n162 = xnode "Motors"() -> ("Sensor"=w833:T3)
                n163 = call-poly <vilib>:"PolySensor.vi"("NXT/EV3"=w834, "Port (Port 1)"=w833) -> ("Scaled Value"=w840:sgl, "NXT/EV3"=w830:T5)  [unwired: 1 in]
                n164 = Greater?(x=w840, y=14.0) -> (0:w839:bool)
                n165 = xnode "Motors"() -> ("Motor"=w832:T4)
                n166 = xnode "Move a Fixed Distance"("Speed 1"=i8 -40, "Distance 1"=w825, "Motors"=w832, "NXT/EV3"=w830) -> ("NXT/EV3"=w829:T5)
                n167 = case shown="False" w839 {
                  tunnel: w838 -> [w857 w861]
                  tunnel: w837 -> [w855 w863]
                  tunnel: [w855 w862] -> w836
                  tunnel: [w856 w861] -> w835
                  tunnel: w829 -> [w854 w860]
                  tunnel: [w854 w859] -> w828
                  frame False {
                    # "No movement for trash"
                    n168 = Increment(x=w857) -> (x+1=w856:i32)
                  }
                  frame True {
                    # "Spin to opaque bay and then return"
                    n169 = Increment(x=w863) -> (x+1=w862:i32)
                    n170 = call "SpinBridge_SubVI.vi"("Motor Spin in"=-114, "BrickReference in"=w860) -> ("BrickReference out"=w859:T5)  [unwired: 9 in]
                  }
                }
                n171 = call <vilib>:"Reset_Timer.vi"("NXT/EV3"=w828, "Timer (Timer 1)"=w826) -> ("NXT/EV3"=w827:T5)  [unwired: 2 in]
              }
              frame True {
              }
            }
          }
        }
        n172 = call-poly <vilib>:"PolyWait.vi"("Time (1 sec)"=sgl 1.0, "NXT/EV3"=w309) -> ("NXT/EV3"=w298:T5)  [unwired: 2 in]
        n173 = xnode "Motors"() -> ("Motor"=w299:T4)
        n174 = xnode "Move Motors"("Power/Speed 1"=25, "Motors"=w299, "NXT/EV3"=w298) -> ("NXT/EV3"=w300:T5)
      }
    }
    "Red Large" <- w258
    "Red Small" <- w257
    "Blue Large" <- w254
    "Blue Small" <- w253
    "White Large" <- w260
    "White Small" <- w259
    "Steel" <- w252
    "HDPE" <- w256
    "Trash" <- w255
    n175 = call-poly <vilib>:"PolySensor.vi"("NXT/EV3"=w248, "Timer (Timer 1)"=w247) -> ("Value (msec)"=w246:u32, "NXT/EV3"=w244:T5)  [unwired: 1 in]
    "Numeric" <- w246
    n176 = Greater?(x=w246, y=u32 30000) -> (0:w249:bool)
    "Process stopped" <- w249
  }
  n177 = Unbundle(w10) -> (w34:i32, w33:i32, w32:i32, w31:i32, w30:i32, w29:i32, w28:i32, w27:i32)
  n178 = xnode "Motors"() -> ("Motor"=w4:T4)
  n179 = xnode "Move Motors"("Power/Speed 1"=i8 0, "Motors"=w4, "NXT/EV3"=w3) -> ("NXT/EV3"=w2:T5)
  n180 = Less Or Equal?(x=w34, y=w26) -> (x <= y?=w58:bool)
  n181 = Less Or Equal?(x=w33, y=w25) -> (x <= y?=w57:bool)
  n182 = Less Or Equal?(x=w32, y=w24) -> (x <= y?=w56:bool)
  n183 = Less Or Equal?(x=w31, y=w23) -> (x <= y?=w55:bool)
  n184 = Less Or Equal?(x=w30, y=w22) -> (x <= y?=w54:bool)
  n185 = Less Or Equal?(x=w29, y=w21) -> (x <= y?=w53:bool)
  n186 = Less Or Equal?(x=w28, y=w20) -> (x <= y?=w52:bool)
  n187 = Less Or Equal?(x=w27, y=w19) -> (x <= y?=w51:bool)
  n188 = Bundle(w58, w57, w56, w55, w54, w53, w52, w51) -> (w50:T6)  [unwired: 1 in]
  n189 = Cluster To Array(cluster=w50) -> (array=w49:bool[])
  n190 = And Array Elements(Boolean array=w49) -> (logical AND=w15:bool)
  n191 = case shown="True" w15 {
    tunnel: w2 -> [w868 w893]
    tunnel: w10 -> [_ w894]
    tunnel: [w867 w883] -> _
    frame False {
      n192 = call-poly <vilib>:"PolySound.vi"("NXT/EV3"=w868) -> ("NXT/EV3"=w867:T5)  [unwired: 3 in]
    }
    frame True {
      # "Each value must be adjusted for the distance the conveyor belt needs to turn"
      # "Dispense Each Marble See:\nDispenseDosage_SubVI"
      n193 = Unbundle(w894) -> (w891:i32, w882:i32, w881:i32, w880:i32, w879:i32, w878:i32, w877:i32, w876:i32)
      n194 = call "DispenseDosage_SubVI.vi"("Numeric 2"=0, "Numeric"=w891, "BrickReference in"=w893) -> ("BrickReference out"=w890:T5)  [unwired: 8 in]
      n195 = call "DispenseDosage_SubVI.vi"("Numeric 2"=0, "Numeric"=w882, "BrickReference in"=w890) -> ("BrickReference out"=w889:T5)  [unwired: 8 in]
      n196 = call "DispenseDosage_SubVI.vi"("Numeric 2"=0, "Numeric"=w881, "BrickReference in"=w889) -> ("BrickReference out"=w888:T5)  [unwired: 8 in]
      n197 = call "DispenseDosage_SubVI.vi"("Numeric 2"=0, "Numeric"=w880, "BrickReference in"=w888) -> ("BrickReference out"=w887:T5)  [unwired: 8 in]
      n198 = call "DispenseDosage_SubVI.vi"("Numeric 2"=0, "Numeric"=w879, "BrickReference in"=w887) -> ("BrickReference out"=w886:T5)  [unwired: 8 in]
      n199 = call "DispenseDosage_SubVI.vi"("Numeric 2"=0, "Numeric"=w878, "BrickReference in"=w886) -> ("BrickReference out"=w885:T5)  [unwired: 8 in]
      n200 = call "DispenseDosage_SubVI.vi"("Numeric 2"=0, "Numeric"=w877, "BrickReference in"=w885) -> ("BrickReference out"=w884:T5)  [unwired: 8 in]
      n201 = call "DispenseDosage_SubVI.vi"("Numeric 2"=0, "Numeric"=w876, "BrickReference in"=w884) -> ("BrickReference out"=w883:T5)  [unwired: 8 in]
    }
  }
